vi "LWXPS_PositionerCorrectorSR1AccelerationGet.vi"(0 "XPS Reference IN":refnum<k24>, 2 "Positioner Name":string, 5 "LabVIEW error IN":errorcluster) -> (8 "XPS Reference OUT":refnum<k24>, 9 "LabVIEW error OUT":errorcluster, 10 "Returned error code":i32, 11 "XPS Error String":string, 12 "Closed loop status":bool, 13 "Jerk compensation gain":dbl, 14 "Proportional gain":dbl, 15 "Integral gain":dbl, 16 "Velocity gain":dbl, 17 "Observer frequency":dbl, 18 "Velocity compensation gain":dbl, 19 "Acceleration compensation gain":dbl)   [LabVIEW 2014]
uses:
  D:/XPSQ8_LabView_Library/Development/Source/Dll/Newport.XPS.CommandInterface.dll
  Dll/Newport.XPS.CommandInterface.dll
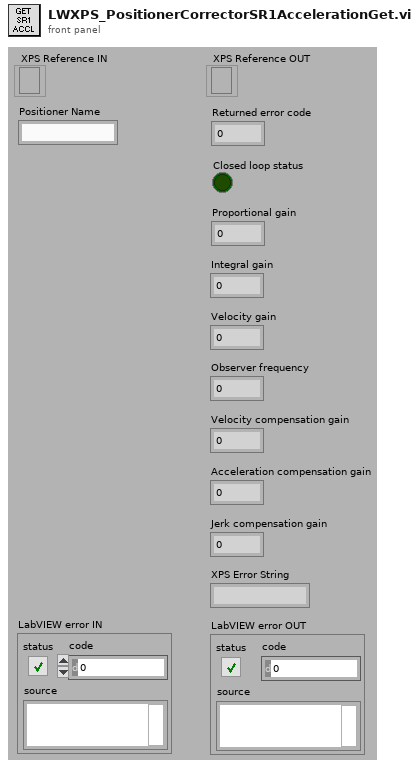
[diagram p1: front panel]
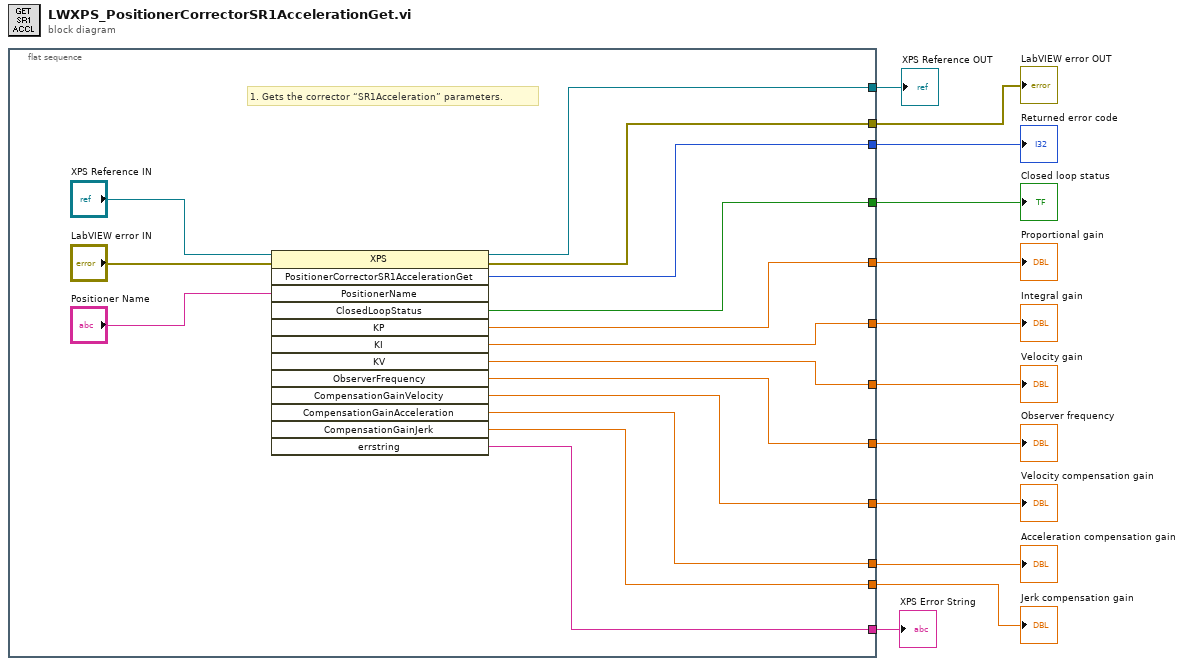
[diagram p0: block diagram]
diagram:
  n1 = flat-sequence {
    tunnel: [w25] -> w12
    tunnel: [w18] -> w11
    tunnel: [w26] -> w10
    tunnel: [w22] -> w9
    tunnel: [w21] -> w8
    tunnel: [w19] -> w7
    tunnel: [w20] -> w6
    tunnel: [w13] -> w5
    tunnel: [w17] -> w2
    tunnel: [w16] -> w3
    tunnel: [w15] -> w1
    tunnel: [w14] -> w4
    frame #0 {
      # "1. Gets the corrector “SR1Acceleration” parameters."
      n2 = invoke class="XPS" method="PositionerCorrectorSR1AccelerationGet"(reference="XPS Reference IN", error in="LabVIEW error IN", "PositionerName"="Positioner Name") -> (reference out=w25:refnum<k24>, error out=w18:errorcluster, "PositionerCorrectorSR1AccelerationGet"=w26:i32, "ClosedLoopStatus"=w17:bool, "KP"=w22:dbl, "KI"=w21:dbl, "KV"=w19:dbl, "ObserverFrequency"=w20:dbl, "CompensationGainVelocity"=w13:dbl, "CompensationGainAcceleration"=w16:dbl, "CompensationGainJerk"=w15:dbl, "errstring"=w14:string)  [unwired: 10 in, 1 out]
    }
  }
  "XPS Error String" <- w4
  "XPS Reference OUT" <- w12
  "LabVIEW error OUT" <- w11
  "Returned error code" <- w10
  "Proportional gain" <- w9
  "Integral gain" <- w8
  "Velocity gain" <- w7
  "Observer frequency" <- w6
  "Velocity compensation gain" <- w5
  "Acceleration compensation gain" <- w3
  "Jerk compensation gain" <- w1
  "Closed loop status" <- w2
